vi "Get Mode.vi"(5 "Ref Mode":refnum<vi>, 6 "Device Found?":bool, 7 "Head Info":string, 8 "error in":errorcluster, 9 "Head Channel":i16, 10 "Pulsar Handle":i16, 11 "OphirFastX (in)":refnum<k7>) -> (0 "error out":errorcluster, 3 "OphirFastX (out)":refnum<k7>)   [LabVIEW 2009]
panel:
  # "Guillaume Plateau - yguig2@yahoo.fr"
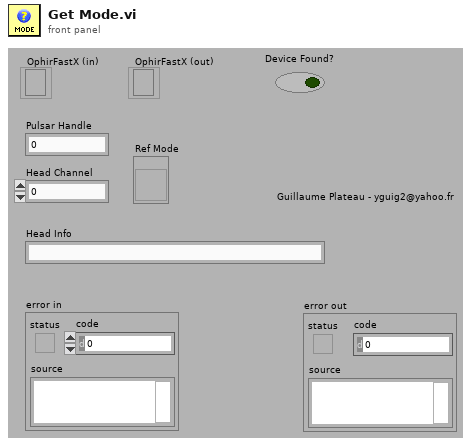
[diagram p1: front panel]
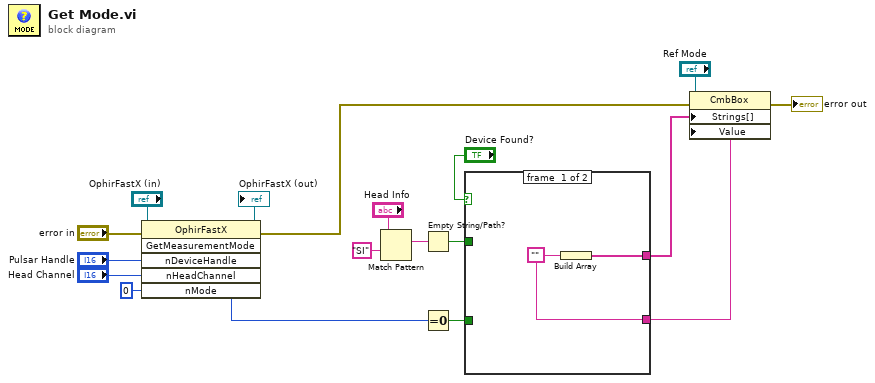
[diagram p0: block diagram]
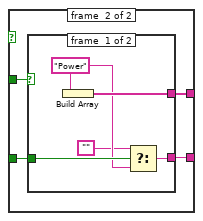
[diagram p2: hidden frame]
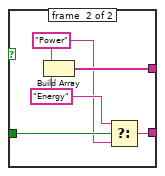
[diagram p3: hidden frame]
diagram:
  n1 = invoke class="OphirFastX" method="GetMeasurementMode"(reference="OphirFastX (in)", error in="error in", "nDeviceHandle"="Pulsar Handle", "nHeadChannel"="Head Channel", "nMode"=i16 0) -> (reference out=→"OphirFastX (out)":refnum<k7>, error out=w4:errorcluster, "nMode"=w16:i16)  [unwired: 1 in, 3 out]
  n2 = Match Pattern(string="Head Info", regular expression="SI") -> (match substring=w12:string)  [unwired: 1 in, 3 out]
  n3 = Empty String/Path?(string/path=w12) -> (empty?=w15:bool)
  n4 = Equal To 0?(x=w16) -> (x = 0?=w17:bool)
  n5 = case shown="True" "Device Found?" {
    tunnel: w15 -> [_ w24]
    tunnel: [w20 w23] -> w3
    tunnel: w17 -> [_ w22]
    tunnel: [w19 w21] -> w2
    frame #0 {
      w19 = ""
      n6 = Build Array(w19) -> (w20:string[])
    }
    frame #1 {
      n7 = case shown="True" w24 {
        tunnel: [w29 w34] -> w23
        tunnel: w22 -> [w28 w33]
        tunnel: [w26 w30] -> w21
        frame #0 {
          w27 = "Power" ("string")
          n8 = Build Array(w27) -> (w29:string[])
          n9 = Select(t="", s=w28, f=w27) -> (s? t:f=w26:string)
        }
        frame #1 {
          w32 = "Energy" ("string")
          w31 = "Power" ("string")
          n10 = Build Array(w31, w32) -> (w34:string[])
          n11 = Select(t=w32, s=w33, f=w31) -> (s? t:f=w30:string)
        }
      }
    }
  }
  n12 = property class="CmbBox"(reference="Ref Mode", error in=w4, "Strings[]"=w3, "Value"=w2) -> (error out=→"error out":errorcluster)  [unwired: 1 out]
